vi "Строку в параметры мишени (SubVI).vi"(2 "Параметры мишени строка":string) -> (8 "Кластер параметров мишени":T1, 13 "Остаток строки параметров":string)   [LabVIEW 2013]
doc: "Преобразует строку считанных из файла параметров мишени в кластер"
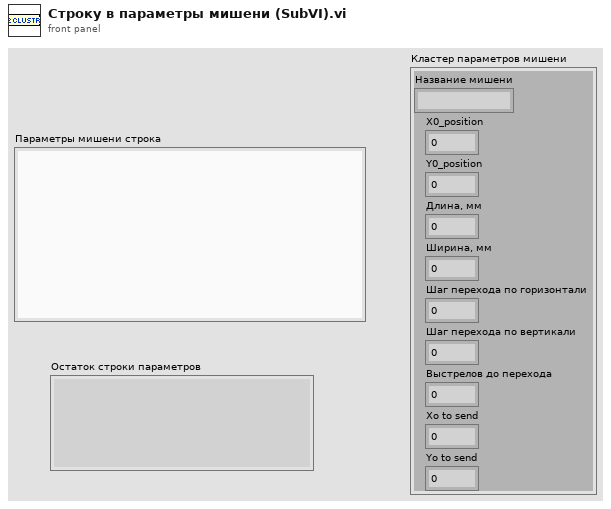
[diagram p1: front panel]
types:
  T1 = cluster{"Название мишени":string, "Х0_position":u16, "Y0_position":u16, "Длина, мм":u16, "Ширина, мм":u16, "Шаг перехода по горизонтали":dbl, "Шаг перехода по вертикали":dbl, "Выстрелов до перехода":u16, "Xo to send ":u16, "Yo to send":u16}
  T2 = cluster{"Параметры мишени строка":string, "default value 1":u16, "default value 1":u16, "default value 1":u16, "default value 1":u16, "default value 1":dbl, "default value 1":dbl, "default value 1":u16, "default value 1":u16, "default value 1":u16}
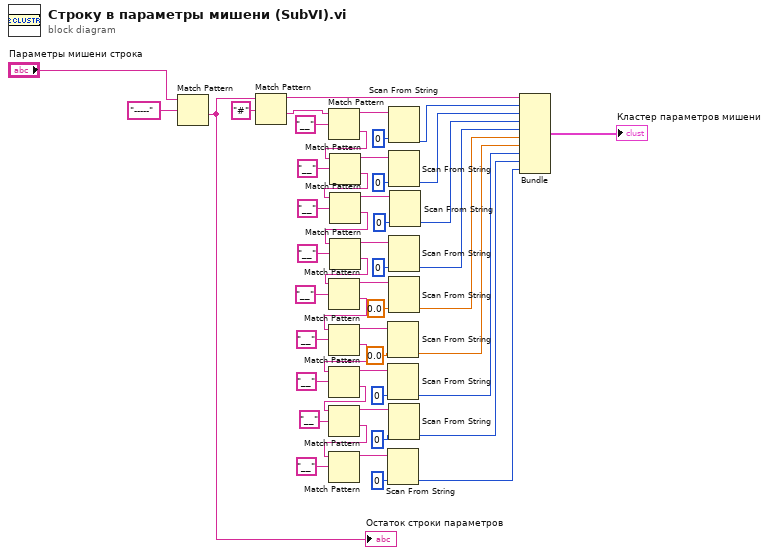
[diagram p0: block diagram]
diagram:
  n1 = Match Pattern(string="Параметры мишени строка", regular expression="-----") -> (after substring=w7:string)  [unwired: 1 in, 3 out]
  "Остаток строки параметров" <- w7
  n2 = Match Pattern(string=w7, regular expression="#" ("delimiter (Tab)")) -> (before substring=w8:string, after substring=w13:string)  [unwired: 1 in, 2 out]
  n3 = Match Pattern(string=w13, regular expression="__" ("delimiter (Tab)")) -> (before substring=w19:string, after substring=w17:string)  [unwired: 1 in, 2 out]
  n4 = Match Pattern(string=w17, regular expression="__" ("delimiter (Tab)")) -> (before substring=w48:string, after substring=w23:string)  [unwired: 1 in, 2 out]
  n5 = Match Pattern(string=w23, regular expression="__" ("delimiter (Tab)")) -> (before substring=w49:string, after substring=w46:string)  [unwired: 1 in, 2 out]
  n6 = Match Pattern(string=w46, regular expression="__" ("delimiter (Tab)")) -> (before substring=w30:string, after substring=w31:string)  [unwired: 1 in, 2 out]
  n7 = Match Pattern(string=w31, regular expression="__" ("delimiter (Tab)")) -> (before substring=w32:string, after substring=w28:string)  [unwired: 1 in, 2 out]
  n8 = Match Pattern(string=w28, regular expression="__" ("delimiter (Tab)")) -> (before substring=w33:string, after substring=w42:string)  [unwired: 1 in, 2 out]
  n9 = Match Pattern(string=w42, regular expression="__" ("delimiter (Tab)")) -> (before substring=w41:string, after substring=w5:string)  [unwired: 1 in, 2 out]
  n10 = Match Pattern(string=w5, regular expression="__" ("delimiter (Tab)")) -> (before substring=w4:string, after substring=w37:string)  [unwired: 1 in, 2 out]
  n11 = Match Pattern(string=w37, regular expression="__" ("delimiter (Tab)")) -> (before substring=w43:string)  [unwired: 1 in, 3 out]
  n12 = Scan From String(input string=w33, default 1=0.0 ("default value 1")) -> (output 1=w35:dbl)  [unwired: 3 in, 3 out]
  n13 = Scan From String(input string=w41, default 1=u16 0 ("default value 1")) -> (output 1=w44:u16)  [unwired: 3 in, 3 out]
  n14 = Scan From String(input string=w43, default 1=u16 0 ("default value 1")) -> (output 1=w45:u16)  [unwired: 3 in, 3 out]
  n15 = Scan From String(input string=w19, default 1=u16 0 ("default value 1")) -> (output 1=w15:u16)  [unwired: 3 in, 3 out]
  n16 = Scan From String(input string=w48, default 1=u16 0 ("default value 1")) -> (output 1=w50:u16)  [unwired: 3 in, 3 out]
  n17 = Scan From String(input string=w30, default 1=u16 0 ("default value 1")) -> (output 1=w24:u16)  [unwired: 3 in, 3 out]
  n18 = Scan From String(input string=w32, default 1=0.0 ("default value 1")) -> (output 1=w34:dbl)  [unwired: 3 in, 3 out]
  n19 = Scan From String(input string=w4, default 1=u16 0 ("default value 1")) -> (output 1=w2:u16)  [unwired: 3 in, 3 out]
  n20 = Scan From String(input string=w49, default 1=u16 0 ("default value 1")) -> (output 1=w51:u16)  [unwired: 3 in, 3 out]
  n21 = Bundle("Параметры мишени строка"=w8, "default value 1"=w15, "default value 1"=w50, "default value 1"=w51, "default value 1"=w24, "default value 1"=w34, "default value 1"=w35, "default value 1"=w44, "default value 1"=w2, "default value 1"=w45) -> (→"Кластер параметров мишени":T2)  [unwired: 1 in]
